vi "Clear Error.vi"(8 "error in (no error)":errorcluster, 11 "configuration session error":T1) -> (0 "error out":errorcluster, 3 "cleared?":bool)   [LabVIEW 2020, in "DSF Core.lvlib" / "Configuration Session.lvclass"]
uses:
  Configuration Session.lvclass
  Errors.ctl
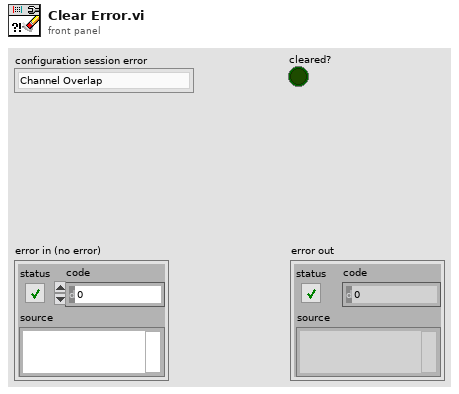
[diagram p1: front panel]
types:
  T1 = typedef "DSF Core.lvlib/Configuration Session.lvclass/Errors.ctl" = enum16{"Channel Overlap", "Invalid Engine Offset", "Invalid JSON"}
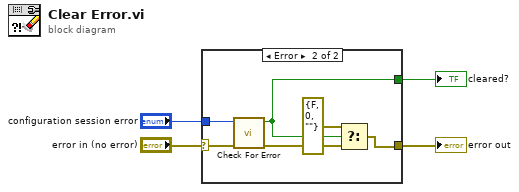
[diagram p0: block diagram]
diagram:
  n1 = case shown="Error" "error in (no error)" {
    selector: "error in (no error)" -> [w5 w11]
    tunnel: "configuration session error" -> [_ w10]
    tunnel: [w5 w7] -> w2
    tunnel: [_ w6] -> w1
    frame No Error {
    }
    frame Error {
      n2 = call "Check For Error.vi"("error in (no error)"=w11, "configuration session error"=w10) -> ("error out"=w9:errorcluster, "is error?"=w6:bool)  [unwired: 8 in]
      n3 = Select(t=errorcluster {"status"=FALSE, "code"=0, "source"=""}, s=w6, f=w9) -> (s? t:f=w7:errorcluster)
    }
  }
  "error out" <- w2
  "cleared?" <- w1
